vi "Init Elec Grid Objects.vi"(7 "Empty Elec Grid Objects":refnum<class "ElectrodeGrid.lvclass">[](array[class]), 8 "error in (no error)":errorcluster, 9 "LG Electrode Grid":bool[][](array[boolean])=[[FALSE, FALSE], [FALSE, FALSE], [FALSE, FALSE]], 10 "SM Electrode Grid":bool[][](array[boolean])=[[FALSE, FALSE, FALSE, FALSE, FALSE, FALSE], [FALSE, FALSE, FALSE, FALSE, FALSE, FALSE], [FALSE, FALSE, FALSE, FALSE, FALSE, FALSE], [FALSE, FALSE, FALSE, FALSE, FALSE, FALSE], [FALSE, FALSE, FALSE, FALSE, FALSE, FALSE], [FALSE, FALSE, FALSE, FALSE, FALSE, FALSE]], 11 "XS Electrode Grid":bool[][](array[boolean])=[[FALSE, FALSE, FALSE], [FALSE, FALSE, FALSE], [FALSE, FALSE, FALSE], [FALSE, FALSE, FALSE], [FALSE, FALSE, FALSE], [FALSE, FALSE, FALSE]]) -> (0 "error out":errorcluster, 3 "Elec Grid Objects":refnum<class "ElectrodeGrid.lvclass">[](array[class]))   [LabVIEW 2017]
doc: "This VI will create 3 instances of electrode grid class. The 3 objects represent XS, SM and LG electrode grids.\n\nObjects are initialized with electrode size, grid and map to HV507 channels of PCB. Modifications to the HV channel map must be made in this VI!\n\nObjects stored and output in an array."
uses:
  Classes/ElectrodeGrid.lvclass
  Classes/ElectrodeGrid.lvclass/ElectrodeGrid.ctl
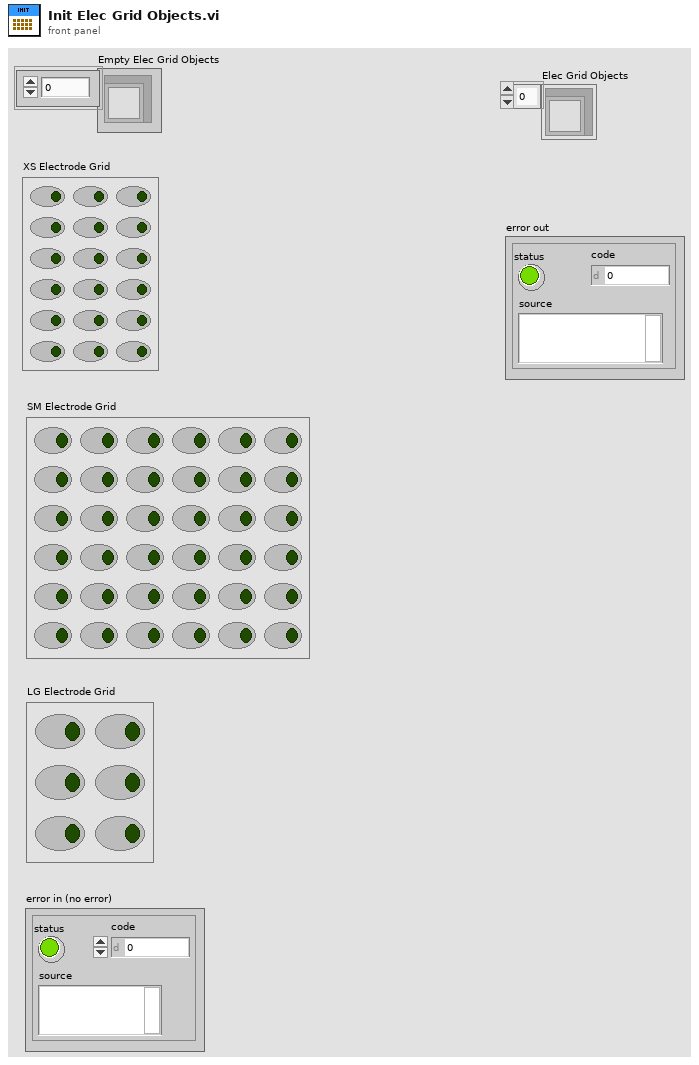
[diagram p1: front panel]
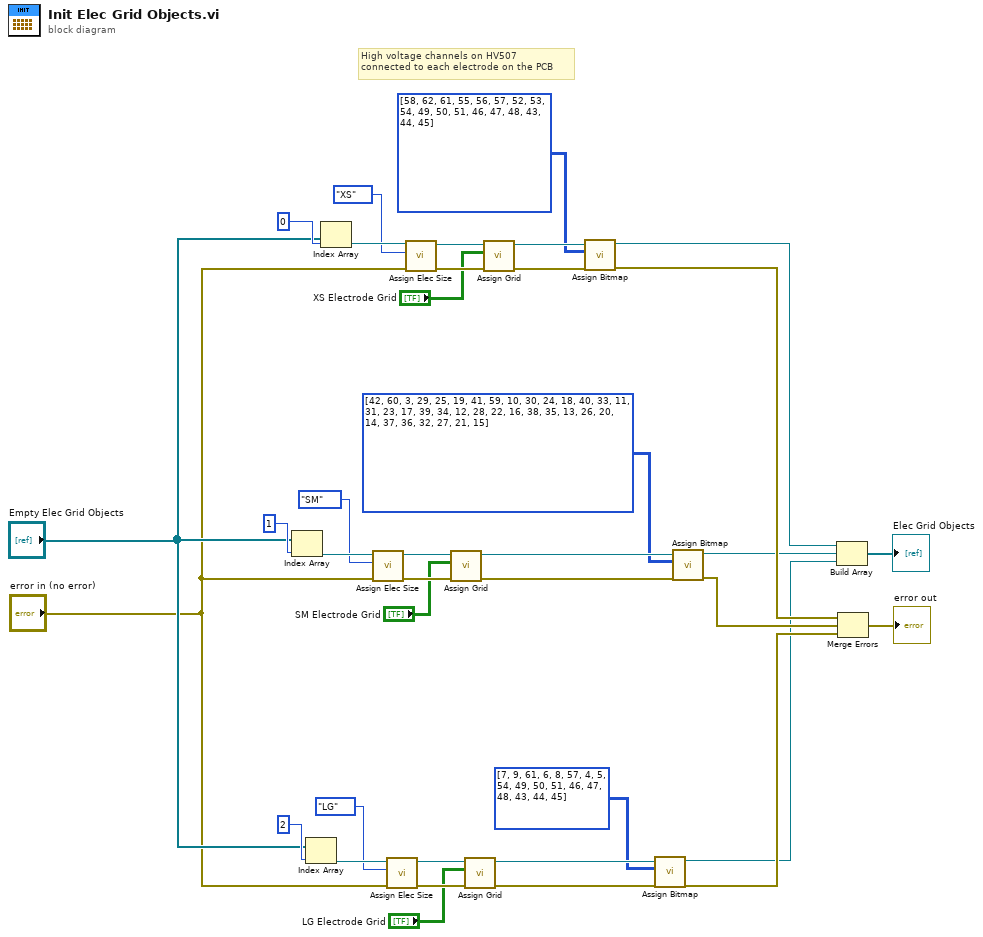
[diagram p0: block diagram]
diagram:
  # "High voltage channels on HV507\nconnected to each electrode on the PCB"
  n1 = Index Array(array="Empty Elec Grid Objects", index=1) -> (element=w22:refnum<class "ElectrodeGrid.lvclass">)
  n2 = Index Array(array="Empty Elec Grid Objects", index=2) -> (element=w14:refnum<class "ElectrodeGrid.lvclass">)
  n3 = Index Array(array="Empty Elec Grid Objects", index=0) -> (element=w36:refnum<class "ElectrodeGrid.lvclass">)
  n4 = call "Assign Elec Size.vi"("error in (no error)"="error in (no error)", "electrode size"=enum16{"XS", "SM", "LG"}."SM", "ElectrodeGrid in"=w22) -> ("error out"=w26:errorcluster, "ElectrodeGrid out"=w27:refnum<class "ElectrodeGrid.lvclass">)  [unwired: 7 in]
  n5 = call "Assign Elec Size.vi"("error in (no error)"="error in (no error)", "electrode size"=enum16{"XS", "SM", "LG"}."LG", "ElectrodeGrid in"=w14) -> ("error out"=w17:errorcluster, "ElectrodeGrid out"=w18:refnum<class "ElectrodeGrid.lvclass">)  [unwired: 7 in]
  n6 = call "Assign Elec Size.vi"("error in (no error)"="error in (no error)", "electrode size"=enum16{"XS", "SM", "LG"}."XS", "ElectrodeGrid in"=w36) -> ("error out"=w33:errorcluster, "ElectrodeGrid out"=w34:refnum<class "ElectrodeGrid.lvclass">)  [unwired: 7 in]
  n7 = call "Assign Grid.vi"("error in (no error)"=w26, "grid"="SM Electrode Grid", "ElectrodeGrid in"=w27) -> ("error out"=w25:errorcluster, "ElectrodeGrid out"=w24:refnum<class "ElectrodeGrid.lvclass">)  [unwired: 7 in]
  n8 = call "Assign Grid.vi"("error in (no error)"=w17, "grid"="LG Electrode Grid", "ElectrodeGrid in"=w18) -> ("error out"=w16:errorcluster, "ElectrodeGrid out"=w15:refnum<class "ElectrodeGrid.lvclass">)  [unwired: 7 in]
  n9 = call "Assign Grid.vi"("error in (no error)"=w33, "grid"="XS Electrode Grid", "ElectrodeGrid in"=w34) -> ("error out"=w31:errorcluster, "ElectrodeGrid out"=w30:refnum<class "ElectrodeGrid.lvclass">)  [unwired: 7 in]
  n10 = call "Assign Bitmap.vi"("error in (no error)"=w31, "bitmap"=u8[][] [[58, 62, 61], [55, 56, 57], [52, 53, 54], [49, 50, 51], [46, 47, 48], [43, 44, 45]], "ElectrodeGrid in"=w30) -> ("error out"=w8:errorcluster, "ElectrodeGrid out"=w4:refnum<class "ElectrodeGrid.lvclass">)  [unwired: 7 in]
  n11 = call "Assign Bitmap.vi"("error in (no error)"=w16, "bitmap"=u8[][] [[7, 9, 61], [6, 8, 57], [4, 5, 54], [49, 50, 51], [46, 47, 48], [43, 44, 45]], "ElectrodeGrid in"=w15) -> ("error out"=w7:errorcluster, "ElectrodeGrid out"=w3:refnum<class "ElectrodeGrid.lvclass">)  [unwired: 7 in]
  n12 = call "Assign Bitmap.vi"("error in (no error)"=w25, "bitmap"=u8[][] [[42, 60, 3, 29, 25, 19], [41, 59, 10, 30, 24, 18], [40, 33, 11, 31, 23, 17], [39, 34, 12, 28, 22, 16], [38, 35, 13, 26, 20, 14], [37, 36, 32, 27, 21, 15]], "ElectrodeGrid in"=w24) -> ("error out"=w9:errorcluster, "ElectrodeGrid out"=w5:refnum<class "ElectrodeGrid.lvclass">)  [unwired: 7 in]
  n13 = Build Array(w4, w5, w3) -> (→"Elec Grid Objects":refnum<class "ElectrodeGrid.lvclass">[])
  n14 = Merge Errors(w8, w9, w7) -> (→"error out":errorcluster)
